vi "Get Summary.vi"(7 "Style":enum16{"Diff", "Plain"}(ring), 8 "error in (no error)":errorcluster, 10 "Item":string, 11 "Result Model by Reference In":refnum<class "Result Model.lvclass">) -> (0 "error out":errorcluster, 2 "Summary":string)   [LabVIEW 2020, in "Result Model.lvclass"]
uses:
  Result Model/Result Model.lvclass
  Result Model/Result Model.lvclass/Result Model.ctl
  Framework/Utilities/Utilities.lvlib
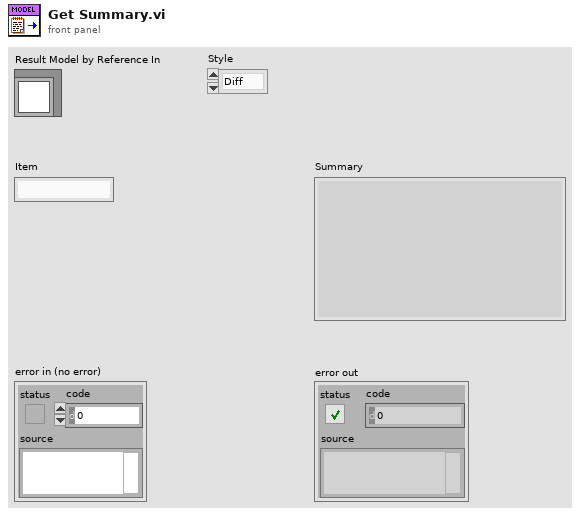
[diagram p1: front panel]
types:
  T1 = typedef "Result.lvlib/Status.ctl" = enum16{"", "Passed", "Failed", "Error", "Skipped", "Setup Error", "Broken", "Teardown Error"}
  T2 = typedef "Result.lvlib/Type.ctl" = enum16{"Test Case", "Test Suite", "Test Run", "Pass", "Fail", "Skip", "Pass if", "Fail if", "Pass if Error", "Fail if Error", "Pass if Equal", "Fail if Equal"}
  T3 = cluster{"Tests":string[], "Run Queue":string[], "Test Statuses":map{string, T1}, "Execution Time":map{string, dbl}, "Assertions":map{string, cluster{"Result Type":T2, "Status":T1, "Description":string, "Data":cluster{"Expected":variant, "Actual":variant, "Delta":variant}}[]}}
  T4 = typedef "Result Model.lvclass/Statistics.ctl" = cluster{"Method Count":u32, "Executed Methods":u32, "Passed Methods":u32, "Failed Methods":u32, "Method Errors":u32, "Skipped Method":u32, "Progress [%]":dbl}
  T5 = map{string, cluster{"Result Type":T2, "Status":T1, "Description":string, "Data":cluster{"Expected":variant, "Actual":variant, "Delta":variant}}[]}
  T6 = cluster{"Result Type":T2, "Status":T1, "Description":string, "Data":cluster{"Expected":variant, "Actual":variant, "Delta":variant}}[]
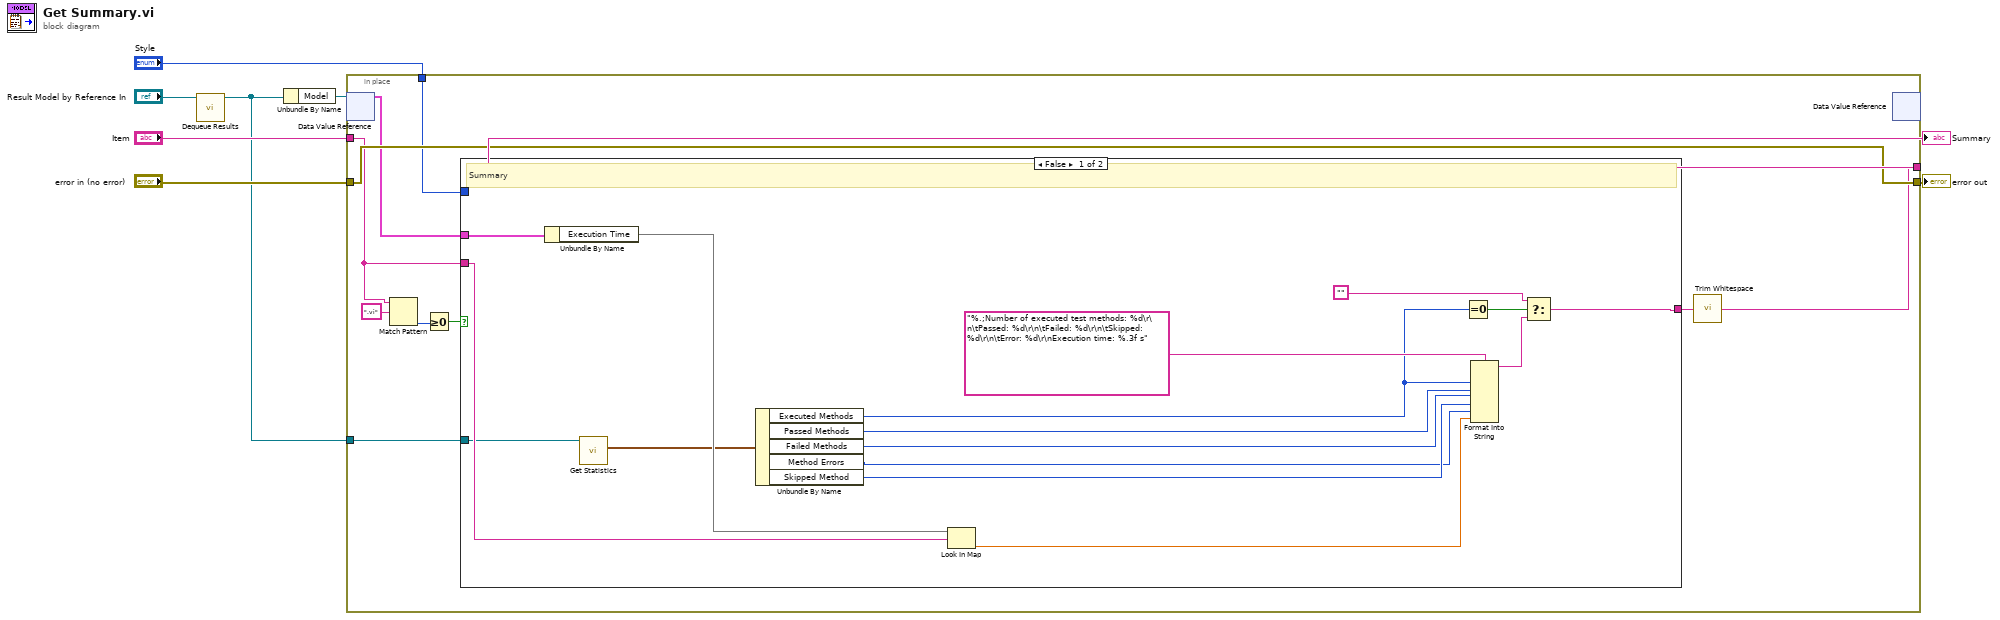
[diagram p0: block diagram]
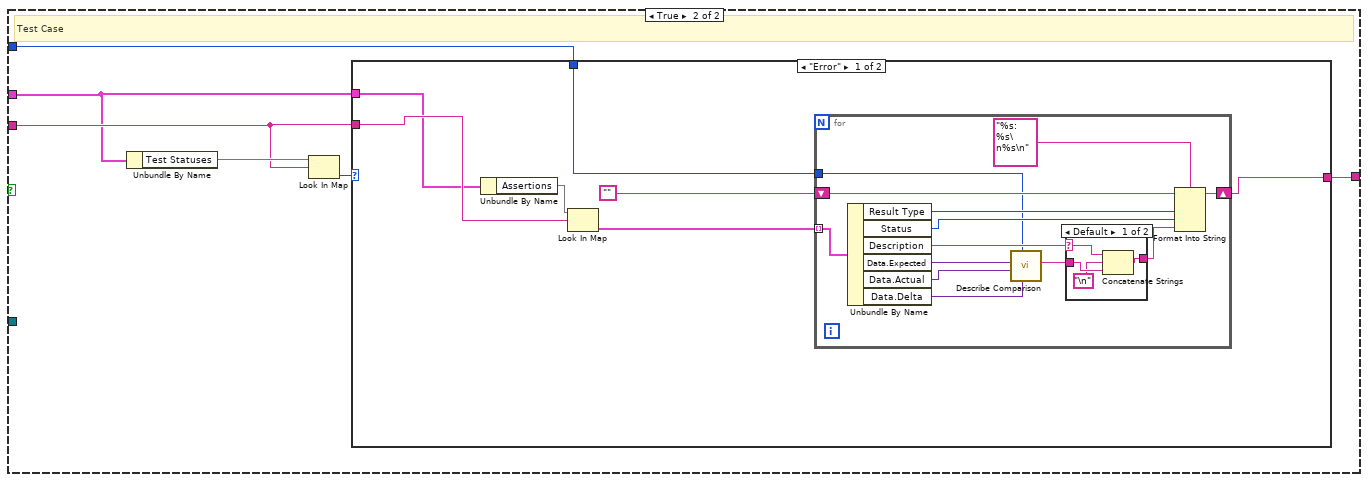
[diagram p2: hidden frame]
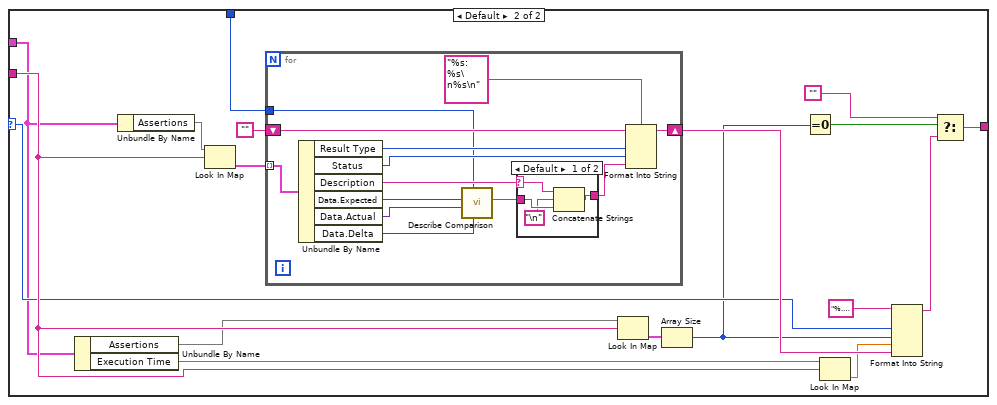
[diagram p4: hidden frame]
diagram:
  n1 = call "Dequeue Results.vi"("Result Model by Reference in"="Result Model by Reference In") -> ("Result Model by Reference out"=w1:refnum<class "Result Model.lvclass">)  [unwired: 10 in]
  n2 = Unbundle By Name(w1) -> ("Model"=w8:refnum<data-value>)
  n3 = in-place {
    in-place-border: "error in (no error)" -> [w18]
    in-place-border: [w18] -> w4
    in-place-border: "Item" -> [w16]
    in-place-border: [w15] -> w3
    in-place-border: "Style" -> [w14]
    in-place-border: w1 -> [w9]
    n4 = in-place-dvr #1(w8) -> (w17:T3)  [unwired: 1 out]
    n5 = Match Pattern(string=w16, regular expression=".vi") -> (offset past match=w11:i32)  [unwired: 1 in, 3 out]
    n6 = Greater Or Equal To 0?(x=w11) -> (x >= 0?=w12:bool)
    n7 = case shown="False" w12 {
      tunnel: w16 -> [w32 w37]
      tunnel: [w28 w39] -> w13
      tunnel: w17 -> [w25 w36]
      tunnel: w14 -> [_ w35]
      tunnel: w9 -> [w19 _]
      frame False {
        # "Summary"
        n8 = Unbundle By Name(w25) -> ("Execution Time"=w26:map{string, dbl})
        n9 = call "Get Statistics.vi"("Result Model in"=w19) -> ("Results"=w24:T4)  [unwired: 9 in, 1 out]
        n10 = Unbundle By Name(w24) -> ("Executed Methods"=w31:u32, "Passed Methods"=w23:u32, "Failed Methods"=w22:u32, "Method Errors"=w20:u32, "Skipped Method"=w21:u32)
        n11 = Look In Map(map=w26, key=w32) -> (value=w33:dbl)  [unwired: 1 in, 1 out]
        n12 = Equal To 0?(x=w31) -> (x = 0?=w30:bool)
        n13 = Format Into String(format string="%.;Number of executed test methods: %d\r\n\tPassed: %d\r\n\tFailed: %d\r\n\tSkipped: %d\r\n\tError: %d\r\nExecution time: %.3f s", w31, w23, w22, w21, w20, w33) -> (resulting string=w29:string)  [unwired: 2 in, 1 out]
        n14 = Select(t="", s=w30, f=w29) -> (s? t:f=w28:string)
      }
      frame True {
        # "Test Case"
        n15 = Unbundle By Name(w36) -> ("Test Statuses"=w38:map{string, T1})
        n16 = Look In Map(map=w38, key=w37) -> (value=w40:T1)  [unwired: 1 in, 1 out]
        n17 = case shown="\"Error\"" w40 {
          selector: w40 -> [_ w74]
          tunnel: [w46 w81] -> w39
          tunnel: w37 -> [w47 w79]
          tunnel: w36 -> [w44 w69]
          tunnel: w35 -> [w45 w70]
          frame "Error" {
            n18 = Unbundle By Name(w44) -> ("Assertions"=w42:T5)
            n19 = Look In Map(map=w42, key=w47) -> (value=w41:T6)  [unwired: 1 in, 1 out]
            n20 = for {
              tunnel: w41 -> [w59] mode=indexing
              shift-right: [w54] -> w46
              shift-left: "" -> [w55]
              tunnel: w45 -> [w48]
              n21 = Unbundle By Name(w59) -> ("Result Type"=w52:T2, "Status"=w51:T1, "Description"=w49:string, "Data.Expected"=w58:variant, "Data.Actual"=w57:variant, "Data.Delta"=w56:variant)
              n22 = call "Describe Comparison.vi"("Delta"=w56, "Style"=w48, "Actual"=w57, "Expected"=w58) -> ("Description"=w53:string)  [unwired: 7 in]
              n23 = case shown="Default" w49 {
                selector: w49 -> [w63 _]
                tunnel: w53 -> [w62 w65]
                tunnel: [w64 w65] -> w50
                frame Default {
                  n24 = Concatenate Strings(w63, "\n", w62) -> (w64:string)
                }
                frame "" {
                }
              }
              n25 = Format Into String(format string="%s: %s\n%s\n", initial string=w55, w52, w51, w50) -> (resulting string=w54:string)  [unwired: 1 in, 1 out]
            }
          }
          frame Default {
            n26 = Unbundle By Name(w69) -> ("Assertions"=w77:T5, "Execution Time"=w78:map{string, dbl})
            n27 = Unbundle By Name(w69) -> ("Assertions"=w67:T5)
            n28 = Look In Map(map=w67, key=w79) -> (value=w66:T6)  [unwired: 1 in, 1 out]
            n29 = for {
              tunnel: w66 -> [w95] mode=indexing
              shift-right: [w90] -> w75
              shift-left: "" -> [w91]
              tunnel: w70 -> [w84]
              n30 = Unbundle By Name(w95) -> ("Result Type"=w88:T2, "Status"=w87:T1, "Description"=w85:string, "Data.Expected"=w94:variant, "Data.Actual"=w93:variant, "Data.Delta"=w92:variant)
              n31 = call "Describe Comparison.vi"("Delta"=w92, "Style"=w84, "Actual"=w93, "Expected"=w94) -> ("Description"=w89:string)  [unwired: 7 in]
              n32 = case shown="Default" w85 {
                selector: w85 -> [w99 _]
                tunnel: w89 -> [w98 w101]
                tunnel: [w100 w101] -> w86
                frame Default {
                  n33 = Concatenate Strings(w99, "\n", w98) -> (w100:string)
                }
                frame "" {
                }
              }
              n34 = Format Into String(format string="%s: %s\n%s\n", initial string=w91, w88, w87, w86) -> (resulting string=w90:string)  [unwired: 1 in, 1 out]
            }
            n35 = Look In Map(map=w77, key=w79) -> (value=w83:T6)  [unwired: 1 in, 1 out]
            n36 = Array Size(array=w83) -> (size(s)=w73:i32)
            n37 = Equal To 0?(x=w73) -> (x = 0?=w82:bool)
            n38 = Look In Map(map=w78, key=w79) -> (value=w72:dbl)  [unwired: 1 in, 1 out]
            n39 = Format Into String(format string="%.;%s, Assertions: %d, Execution time: %.3f \n\n%s", w74, w73, w72, w75) -> (resulting string=w76:string)  [unwired: 2 in, 1 out]
            n40 = Select(t="", s=w82, f=w76) -> (s? t:f=w81:string)
          }
        }
      }
    }
    n41 = call <vilib>:"Trim Whitespace.vi"("string"=w13) -> ("trimmed string"=w15:string)  [unwired: 1 in]
    n42 = in-place-dvr #1() -> ()  [unwired: 1 in, 2 out]
  }
  "Summary" <- w3
  "error out" <- w4
